vi "Get Endpoints from Switches JSON.vi"(8 "error in (no error)":errorcluster, 10 "topology":string, 11 "switches json":string) -> (0 "error out":errorcluster, 3 "endpoints":string[](array[string]))   [LabVIEW 2017, in "SLSC Switch Examples.lvlib"]
uses:
  SLSC Switch Examples.lvlib
  <vilib>/SLSC_Switch/Initialize with Topology (Simulate).vi
  <vilib>/SLSC_Switch/SLSC Switch.lvlib
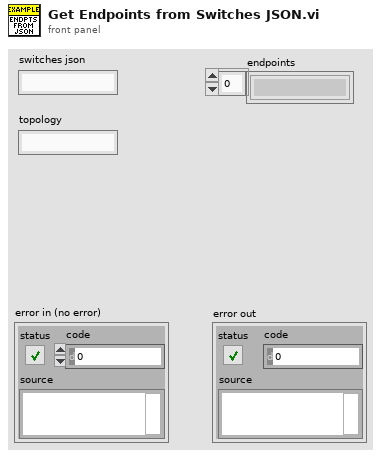
[diagram p1: front panel]
types:
  T1 = typedef "nislscslSession.ctl" = refnum<k20>
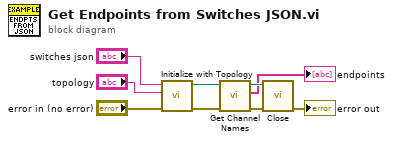
[diagram p0: block diagram]
diagram:
  n1 = call-poly <vilib>:"Initialize with Topology.vi"("error in (no error)"="error in (no error)", "topology"="topology", "switches json"="switches json") -> ("error out"=w5:errorcluster, "session out"=w6:T1)  [unwired: 7 in]
  n2 = call <vilib>:"Get Channel Names.vi"("error in (no error)"=w5, "session in"=w6) -> ("error out"=w3:errorcluster, "channel names"=→"endpoints":string[], "session out"=w4:T1)  [unwired: 7 in]
  n3 = call <vilib>:"Close.vi"("error in (no error)"=w3, "session in"=w4) -> ("error out"=→"error out":errorcluster)  [unwired: 9 in]
